vi "Configure Gate View.vi"   [LabVIEW 2020, in "Anritsu Signal Analyzer Series.lvlib"]
doc: "Configures the Gate View settings."
uses:
  Anritsu Signal Analyzer Series.lvlib
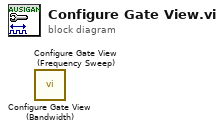
[diagram p0: block diagram]
diagram:
  n1 = call "Configure Gate View (Bandwidth).vi"() -> ()  [unwired: 14 in, 2 out]
  n2 = call "Configure Gate View (Frequency Sweep).vi"() -> ()  [unwired: 14 in, 2 out]
